vi "Send Element Touched event.vi"(8 "error in (no error)":errorcluster, 10 "event data":T1, 11 "D_Datagrid in":refnum<class "D_Datagrid.lvclass">) -> (0 "error out":errorcluster, 3 "D_Datagrid out":refnum<class "D_Datagrid.lvclass">)   [LabVIEW 2020, in "D Datagrid Library.lvlib" / "D_Datagrid.lvclass"]
doc: "Sends the Element Touched event. This VI is Dynamic Dispatch, so it can be overridden to create custom behavior."
uses:
  D_Datagrid.lvclass
  D_Datagrid.lvclass/D_Datagrid.ctl
  DatagridElement/DatagridElement.lvclass
  D Datagrid Update Element.ctl
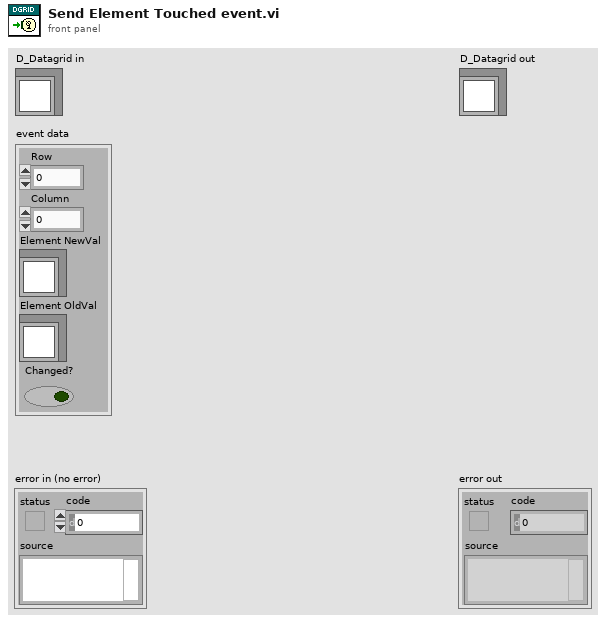
[diagram p1: front panel]
types:
  T1 = typedef "D Datagrid Library.lvlib/D_Datagrid.lvclass/D Datagrid Update Element.ctl" = cluster{"Row":i32, "Column":i32, "Element NewVal":refnum<class "DatagridElement.lvclass">, "Element OldVal":refnum<class "DatagridElement.lvclass">, "Changed?":bool}
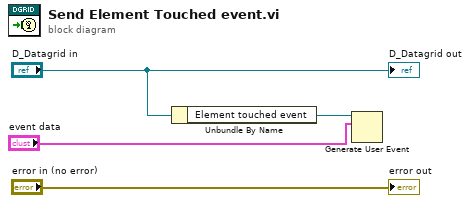
[diagram p0: block diagram]
diagram:
  n1 = Unbundle By Name("D_Datagrid in") -> ("Element touched event"=w4:refnum<user-event>)
  n2 = Generate User Event(user event=w4, event data cluster="event data") -> ()  [unwired: 2 in, 2 out]
  "error out" <- "error in (no error)"
  "D_Datagrid out" <- "D_Datagrid in"
